vi "VI Server_Set ComboBox by Item Selected.vi"(7 "Label":string, 8 "error in":errorcluster, 9 "Item Selected":string, 11 "VI Server Cluster":T1) -> (0 "error out":errorcluster, 1 "ComboBoxRef":refnum<vi>, 3 "VI Server Cluster.DUP":T1)   [LabVIEW 2020, in "VI Server Toolkit LV2013.lvlib"]
doc: "Sets Menu Ring value/selection by the item name."
uses:
  VI Server Toolkit LV2013.lvlib
  VI Server_TypeDefs/VI Server_RefsCluster.ctl
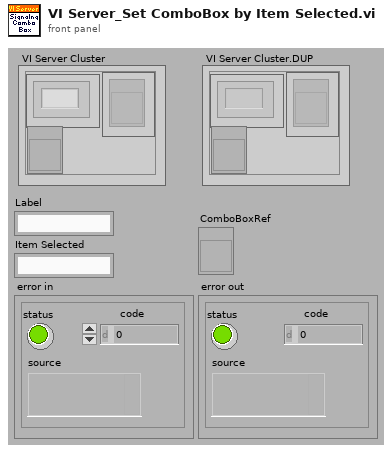
[diagram p1: front panel]
types:
  T1 = typedef "VI Server_RefsCluster.ctl" = cluster{"Labels":string[], "Refs":refnum<vi>[], "VI Ref":refnum<vi>}
  T2 = typedef "LVComboBoxStrsAndValuesArrayTypeDef.ctl" = cluster{"String":string, "Value":string}[]
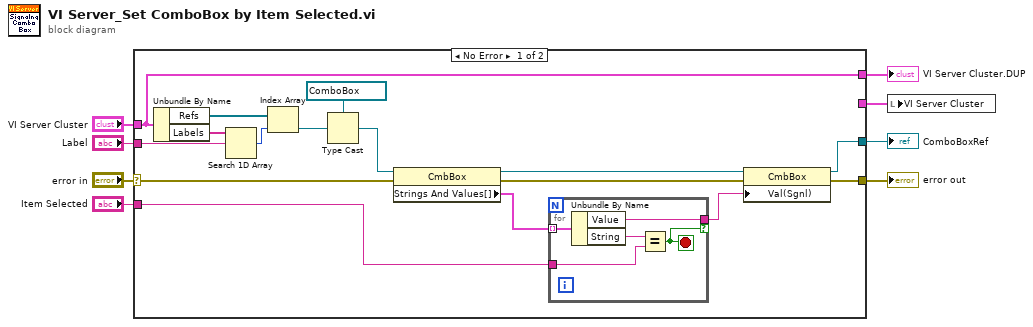
[diagram p0: block diagram]
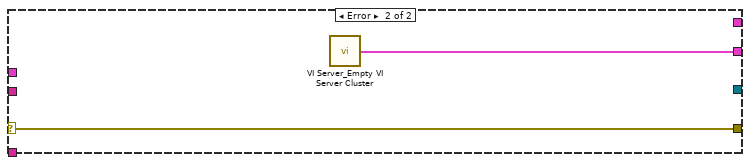
[diagram p2: hidden frame]
diagram:
  n1 = case shown="No Error" "error in" {
    selector: "error in" -> [w18 w31]
    tunnel: "Label" -> [w23 _]
    tunnel: "VI Server Cluster" -> [w16 _]
    tunnel: [w12 w31] -> w8
    tunnel: [w10 _] -> w3
    tunnel: "Item Selected" -> [w14 _]
    tunnel: [w16 _] -> w2
    tunnel: [_ w30] -> w1
    frame No Error {
      n2 = Unbundle By Name(w16) -> ("Refs"=w21:refnum<vi>[], "Labels"=w24:string[])
      n3 = Search 1D Array(1D array=w24, element=w23) -> (index of element=w22:i32)  [unwired: 1 out]
      n4 = Index Array(array=w21, index=w22) -> (element=w20:refnum<vi>)
      n5 = Type Cast(type=refnum<vi> refnum ("Combo Box"), x=w20) -> (*(type *) &x=w17:refnum<vi>)
      n6 = property class="CmbBox"(reference=w17, error in=w18) -> (reference out=w11:refnum<vi>, error out=w13:errorcluster, "Strings And Values[]"=w15:T2)
      n7 = for {
        tunnel: w15 -> [w29] mode=indexing
        tunnel: w14 -> [w27]
        tunnel: [w26] -> w9 if=w25
        stop <- w25 stop-if-true
        n8 = Unbundle By Name(w29) -> ("Value"=w26:string, "String"=w28:string)
        n9 = Equal?(x=w28, y=w27) -> (x = y?=w25:bool)
      }
      n10 = property class="CmbBox"(reference=w11, error in=w13, "Val(Sgnl)"=w9) -> (reference out=w10:refnum<vi>, error out=w12:errorcluster)
    }
    frame Error {
      n11 = call "VI Server_Empty VI Server Cluster.vi"() -> ("VI Server Cluster"=w30:T1)  [unwired: 7 in]
    }
  }
  "error out" <- w8
  "VI Server Cluster.DUP" <- w2
  "ComboBoxRef" <- w3
  n12 = local write "VI Server Cluster"(w1) -> ()
